vi "Set Grating.vi"(8 "error in (no error)":errorcluster, 9 "Wait for Reply?":bool=TRUE, 10 "Grating ID":u32, 11 "Simulated in":refnum<class "Simulated.lvclass">) -> (0 "error out":errorcluster, 2 "Grating ID out":u32, 3 "Simulated out":refnum<class "Simulated.lvclass">)   [LabVIEW 2019, in "Simulated.lvclass"]
uses:
  Simulated.lvclass
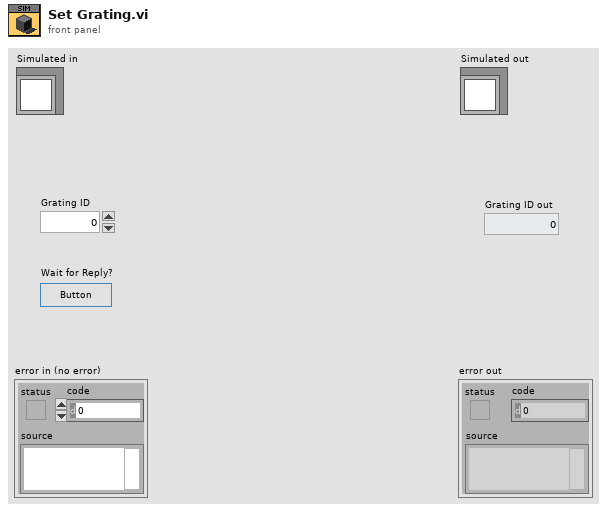
[diagram p1: front panel]
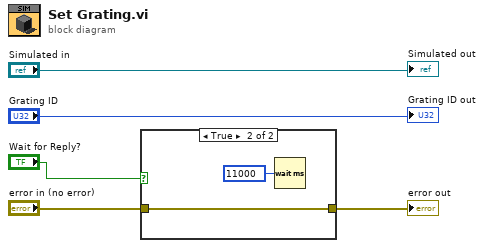
[diagram p0: block diagram]
diagram:
  n1 = case shown="True" "Wait for Reply?" {
    tunnel: "error in (no error)" -> [w6 w8]
    tunnel: [w6 w8] -> w4
    frame False {
    }
    frame True {
      n2 = Wait (ms)(milliseconds to wait=u32 11000) -> ()  [unwired: 1 out]
    }
  }
  "error out" <- w4
  "Simulated out" <- "Simulated in"
  "Grating ID out" <- "Grating ID"
